vi "Read Export Operation Errors.vi"(8 "Error In":errorcluster, 11 "Export in":refnum<class "Export.lvclass">) -> (0 "Error Out":errorcluster, 2 "Export Operation Errors":errorcluster, 3 "Export out":refnum<class "Export.lvclass">)   [LabVIEW 2017, in "CL_G3_VIComponentBuilder.lvlib" / "Export.lvclass"]
uses:
  Export.lvclass
  Export.lvclass/Export.ctl
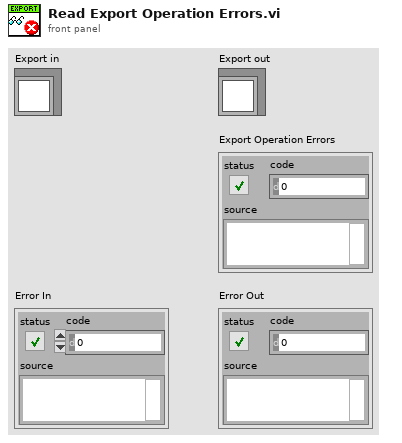
[diagram p1: front panel]
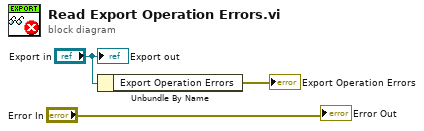
[diagram p0: block diagram]
diagram:
  n1 = Unbundle By Name("Export in") -> ("Export Operation Errors"=→"Export Operation Errors":errorcluster)
  "Export out" <- "Export in"
  "Error Out" <- "Error In"
